vi "gradient_fo.vi"(1 "q_input":dbl[](array[numeric]), 2 "Object cluster":T1) -> (0 "Gradient of fo":dbl[](array[numeric]))   [LabVIEW 2019]
panel:
  # "input : object cluster\n             q_input"
  # "output : gradient_fo, \n               vector"
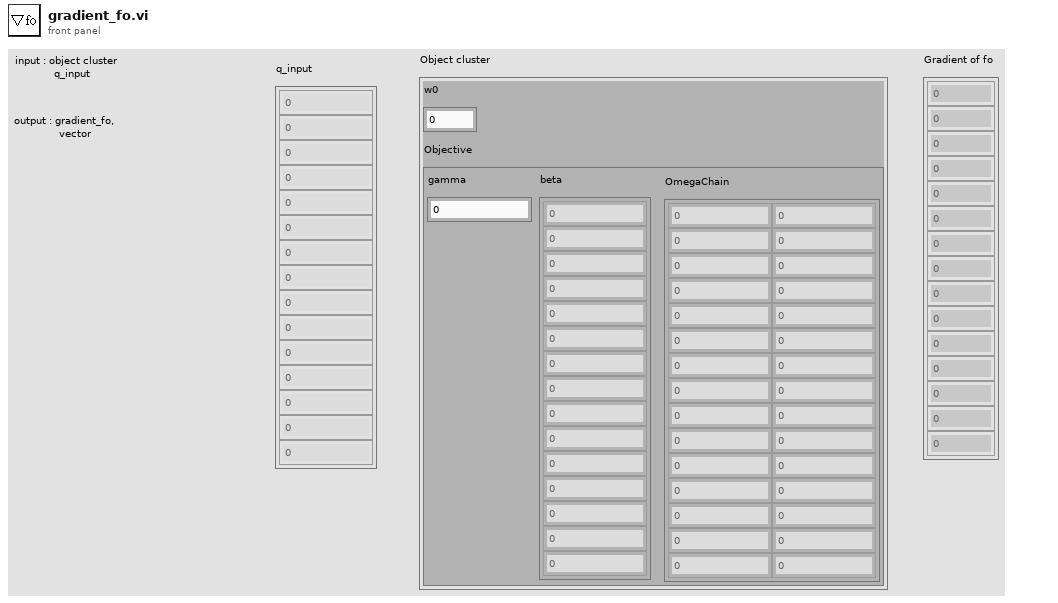
[diagram p1: front panel]
types:
  T1 = cluster{"w0":dbl, "Objective":cluster{"beta":dbl[], "gamma":dbl, "OmegaChain":dbl[][]}}
  T2 = cluster{"beta":dbl[], "gamma":dbl, "OmegaChain":dbl[][]}
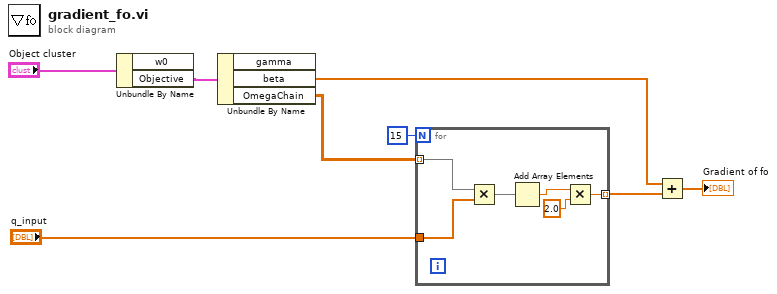
[diagram p0: block diagram]
diagram:
  n1 = Unbundle By Name("Object cluster") -> ("Objective"=w6:T2)  [unwired: 1 out]
  n2 = Unbundle By Name(w6) -> ("beta"=w2:dbl[], "OmegaChain"=w4:dbl[][])  [unwired: 1 out]
  n3 = for {
    N: 15 -> [_]
    tunnel: "q_input" -> [w12]
    tunnel: [w10] -> w3 mode=indexing
    tunnel: w4 -> [w11] mode=indexing
    n4 = Multiply(x=w11, y=w12) -> (x*y=w14:dbl[])
    n5 = Add Array Elements(numeric array=w14) -> (sum=w13:dbl)
    n6 = Multiply(x=w13, y=2.0) -> (x*y=w10:dbl)
  }
  n7 = Add(x=w2, y=w3) -> (x+y=→"Gradient of fo":dbl[])
